vi "xijk_write_fifo_search_list.vi"(5 "file path cluster in":T1, 6 "Emission filter 2":path, 7 "Excitation filter 1":path, 8 "Dichroic filter 2":path, 9 "Excitation filter 2":path, 10 "Emission filter 1":path, 11 "Dichroic filter 1":path) -> (3 "file path cluster out":T1)   [LabVIEW 2009]
uses:
  Type Def/filepath.ctl
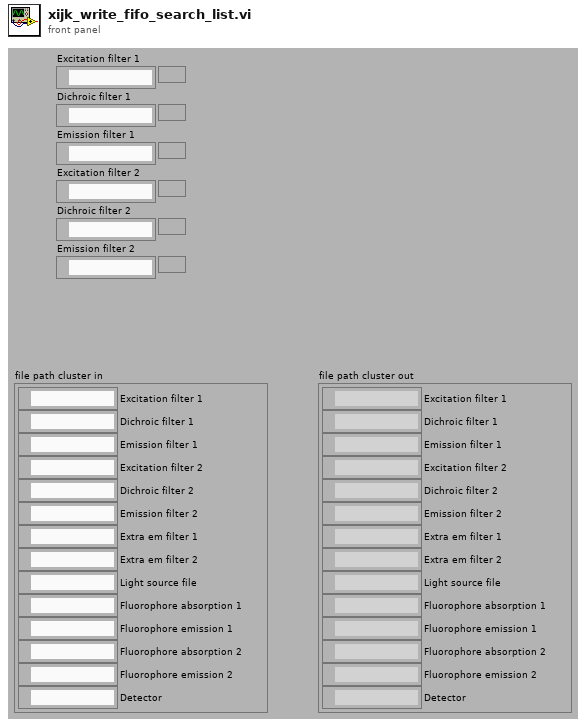
[diagram p1: front panel]
types:
  T1 = typedef "filepath.ctl" = cluster{"Excitation filter 1":path, "Dichroic filter 1":path, "Emission filter 1":path, "Excitation filter 2":path, "Dichroic filter 2":path, "Emission filter 2":path, "Extra em filter 1":path, "Extra em filter 2":path, "Light source file":path, "Fluorophore absorption 1":path, "Fluorophore emission 1":path, "Fluorophore absorption 2":path, "Fluorophore emission 2":path, "Detector":path}
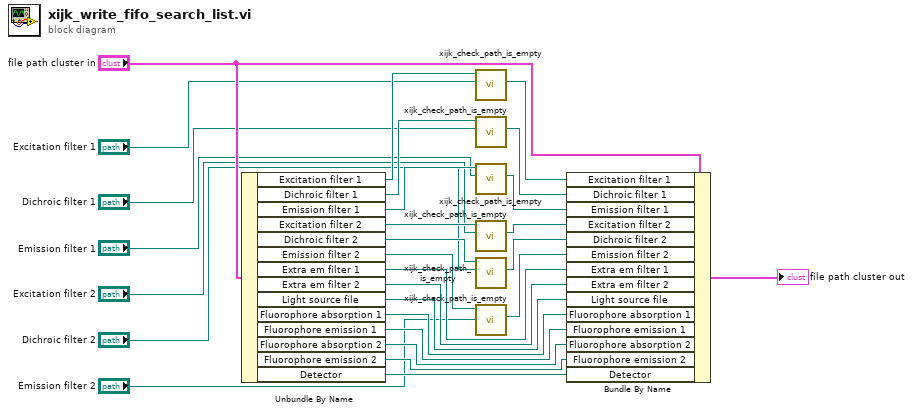
[diagram p0: block diagram]
diagram:
  n1 = Unbundle By Name("file path cluster in") -> ("Excitation filter 1"=w26:path, "Dichroic filter 1"=w25:path, "Emission filter 1"=w24:path, "Excitation filter 2"=w23:path, "Dichroic filter 2"=w21:path, "Emission filter 2"=w22:path, "Extra em filter 1"=w15:path, "Extra em filter 2"=w14:path, "Light source file"=w13:path, "Fluorophore absorption 1"=w12:path, "Fluorophore emission 1"=w11:path, "Fluorophore absorption 2"=w10:path, "Fluorophore emission 2"=w9:path, "Detector"=w8:path)
  n2 = call "xijk_check_path_is_empty.vi"("Excitation filter 2"="Excitation filter 1", "Path"=w26) -> ("Excitation filter 1"=w27:path)  [unwired: 9 in]
  n3 = call "xijk_check_path_is_empty.vi"("Excitation filter 2"="Dichroic filter 1", "Path"=w25) -> ("Excitation filter 1"=w20:path)  [unwired: 9 in]
  n4 = call "xijk_check_path_is_empty.vi"("Excitation filter 2"="Emission filter 1", "Path"=w24) -> ("Excitation filter 1"=w19:path)  [unwired: 9 in]
  n5 = call "xijk_check_path_is_empty.vi"("Excitation filter 2"="Excitation filter 2", "Path"=w23) -> ("Excitation filter 1"=w18:path)  [unwired: 9 in]
  n6 = call "xijk_check_path_is_empty.vi"("Excitation filter 2"="Dichroic filter 2", "Path"=w21) -> ("Excitation filter 1"=w17:path)  [unwired: 9 in]
  n7 = call "xijk_check_path_is_empty.vi"("Excitation filter 2"="Emission filter 2", "Path"=w22) -> ("Excitation filter 1"=w16:path)  [unwired: 9 in]
  n8 = Bundle By Name(cluster="file path cluster in", "Excitation filter 1"=w27, "Dichroic filter 1"=w20, "Emission filter 1"=w19, "Excitation filter 2"=w18, "Dichroic filter 2"=w17, "Emission filter 2"=w16, "Extra em filter 1"=w15, "Extra em filter 2"=w14, "Light source file"=w13, "Fluorophore absorption 1"=w12, "Fluorophore emission 1"=w11, "Fluorophore absorption 2"=w10, "Fluorophore emission 2"=w9, "Detector"=w8) -> (→"file path cluster out":T1)
